vi "Save BG Image Error.vi"(11 "Camera Name":string) -> ()   [LabVIEW 2014, in "HIJ IMAQdx Display.lvlib" / "HIJ IMAQdx Display.lvclass"]
uses:
  HIJ IMAQdx Display.lvclass
panel:
  out "String":string
  in  "OK Button":bool
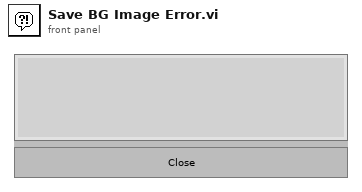
[diagram p1: front panel]
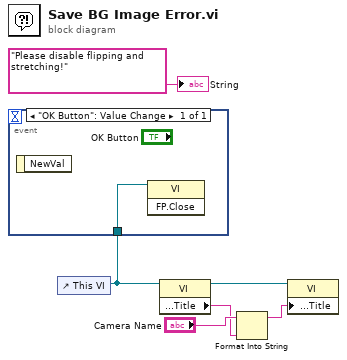
[diagram p0: block diagram]
diagram:
  n1 = control-ref of="This VI"() -> (w5:refnum<vi>)
  n2 = event shown="[0] \"OK Button\": Value Change" {
    selector: _ -> [_]
    dyn-events: _ -> [_]
    timeout: _ -> [_]
    tunnel: w5 -> [w7]
    event "OK Button": Value Change {
      n3 = event-data() -> ()  [unwired: 1 in, 1 out]
      n4 = invoke class="VI" method="FP.Close"(reference=w7) -> ()  [unwired: 2 in, 3 out]
    }
  }
  n5 = property class="VI"(reference=w5) -> (reference out=w4:refnum<vi>, "Front Panel.Title"=w2:string)  [unwired: 1 in, 1 out]
  n6 = Format Into String(initial string="Camera Name", w2) -> (resulting string=w1:string)  [unwired: 2 in, 1 out]
  n7 = property class="VI"(reference=w4, "Front Panel.Title"=w1) -> ()  [unwired: 1 in, 2 out]
  "String" <- "Please disable flipping and stretching!" ("String")
